vi "Configure Measurement Characteristics (Baseband Noise).vi"(0 "VISA resource name":refnum<visa-resource-name>, 1 "Measurement Quality (1: Normal)":u16(ring)=1 items=["Fast", "Normal"], 7 "Data Format (1: dBV/Hz)":u16(ring)=1 items=["dBm/Hz", "dBV/Hz"], 11 "error in (no error)":errorcluster) -> (4 "VISA resource name out":refnum<visa-resource-name>, 15 "error out":errorcluster)   [LabVIEW 2011, in "Agilent E5052X.lvlib"]
doc: "Configures initial settings for Baseband Noise measurement. \n\n<b>Note:</b> \n\n1) Baseband Noise measurement is not available on the Agilent E5052A Signal Source Analyzer.\n\n2) This VI must be called first before calling \"Configure Measurement(Baseband)\" VI."
uses:
  Agilent E5052X.lvlib
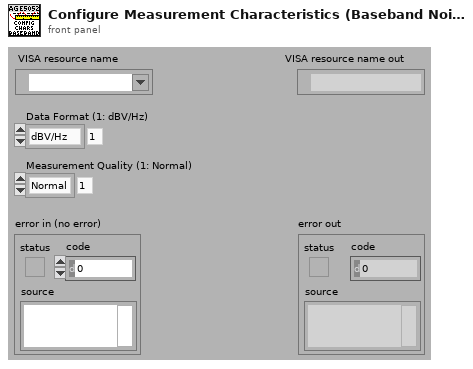
[diagram p1: front panel]
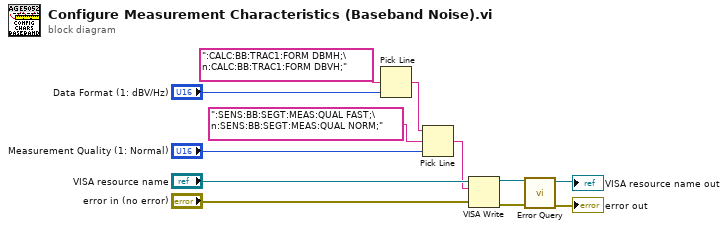
[diagram p0: block diagram]
diagram:
  n1 = Pick Line(multi-line string=":CALC:BB:TRAC1:FORM DBMH;\n:CALC:BB:TRAC1:FORM DBVH;", line index="Data Format (1: dBV/Hz)") -> (output string=w2:string)  [unwired: 1 in]
  n2 = Pick Line(string ("")=w2, multi-line string=":SENS:BB:SEGT:MEAS:QUAL FAST;\n:SENS:BB:SEGT:MEAS:QUAL NORM;", line index="Measurement Quality (1: Normal)") -> (output string=w1:string)
  n3 = VISA Write(VISA resource name="VISA resource name", write buffer=w1, error in (no error)="error in (no error)") -> (VISA resource name out=w12:refnum<visa-resource-name>, error out=w11:errorcluster)  [unwired: 1 out]
  n4 = call "Error Query.vi"("error in (no error)"=w11, "VISA resource name"=w12) -> ("error out"=→"error out":errorcluster, "VISA resource name out"=→"VISA resource name out":refnum<visa-resource-name>)  [unwired: 6 in, 2 out]
